vi "CameraParams_AE.vi"(2 "Action":T2, 7 "Camera Parameters":T1 {"Master Gain" scale=0.067..100.0; "Black Level Offset" scale=0.067..255.0; "Exposure Time (ms)" scale=0.067..71.0; "Frame Rate" scale=5.0..14.0; "Pixel Clock" scale=5.0..43.0}, 11 "Save Path":path=path "Not A Path") -> (8 "Camera Parameters Out":T1 {"Master Gain" scale=0.067..100.0; "Black Level Offset" scale=0.067..255.0; "Exposure Time (ms)" scale=0.067..71.0; "Frame Rate" scale=5.0..14.0; "Pixel Clock" scale=5.0..43.0}, 15 "Save Path Out":path)   [LabVIEW 2016]
uses:
  Controls/Camera Parameters.ctl
  Controls/StandardAction.ctl
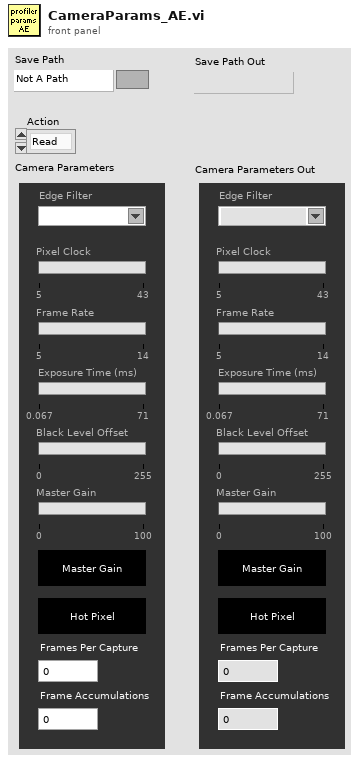
[diagram p1: front panel]
types:
  T1 = typedef "Camera Parameters.ctl" = cluster{"Edge Filter":string, "Pixel Clock":i32, "Frame Rate":dbl, "Exposure Time (ms)":dbl, "Black Level Offset":i32, "Master Gain":i32, "Master Gain Bool":bool, "Hot Pixel Correction":bool, "Frames Per Capture":u32, "Frame Accumulations":u32}
  T2 = typedef "StandardAction.ctl" = enum16{"Read", "Write"}
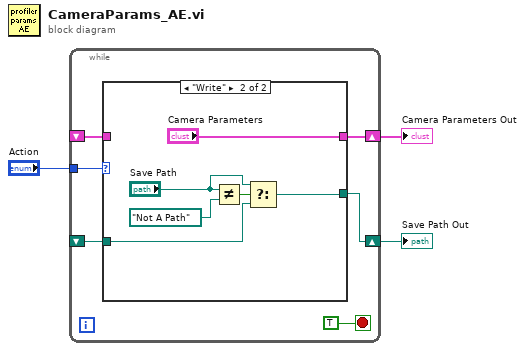
[diagram p0: block diagram]
diagram:
  n1 = while {
    shift-right: [w7] -> w2
    shift-left: _ -> [w6]
    tunnel: "Action" -> [w8]
    shift-right: [w5] -> w1
    shift-left: _ -> [w4]
    stop <- TRUE stop-if-true
    n2 = case shown="\"Write\"" w8 {
      tunnel: [w11 "Camera Parameters"] -> w7
      tunnel: w6 -> [w11 _]
      tunnel: [w10 w13] -> w5
      tunnel: w4 -> [w10 w12]
      frame "Read", Default {
      }
      frame "Write" {
        n3 = Not Equal?(x="Save Path", y=path "Not A Path" ("Save Path")) -> (x != y?=w15:bool)
        n4 = Select(t="Save Path", s=w15, f=w12) -> (s? t:f=w13:path)
      }
    }
  }
  "Camera Parameters Out" <- w2
  "Save Path Out" <- w1
